vi "Water tank Sequence (1).vi"() -> ()   [LabVIEW 2023]
panel:
  out "Overhead Tank Chart":dbl(graph)
  out "Domestic Supply Chart":dbl(graph)
  out "Underground Tank Chart":dbl(graph)
  in  "Domestic Supply":bool
  in  "Overhead Tank":bool
  out "Domestic Supply":dbl(slide) scale=0.0..1000.0
  in  "Underground Tank":bool
  out "Overhead Tank":dbl(slide) scale=0.0..1000.0
  out "Underground Tank":dbl(slide) scale=0.0..5000.0
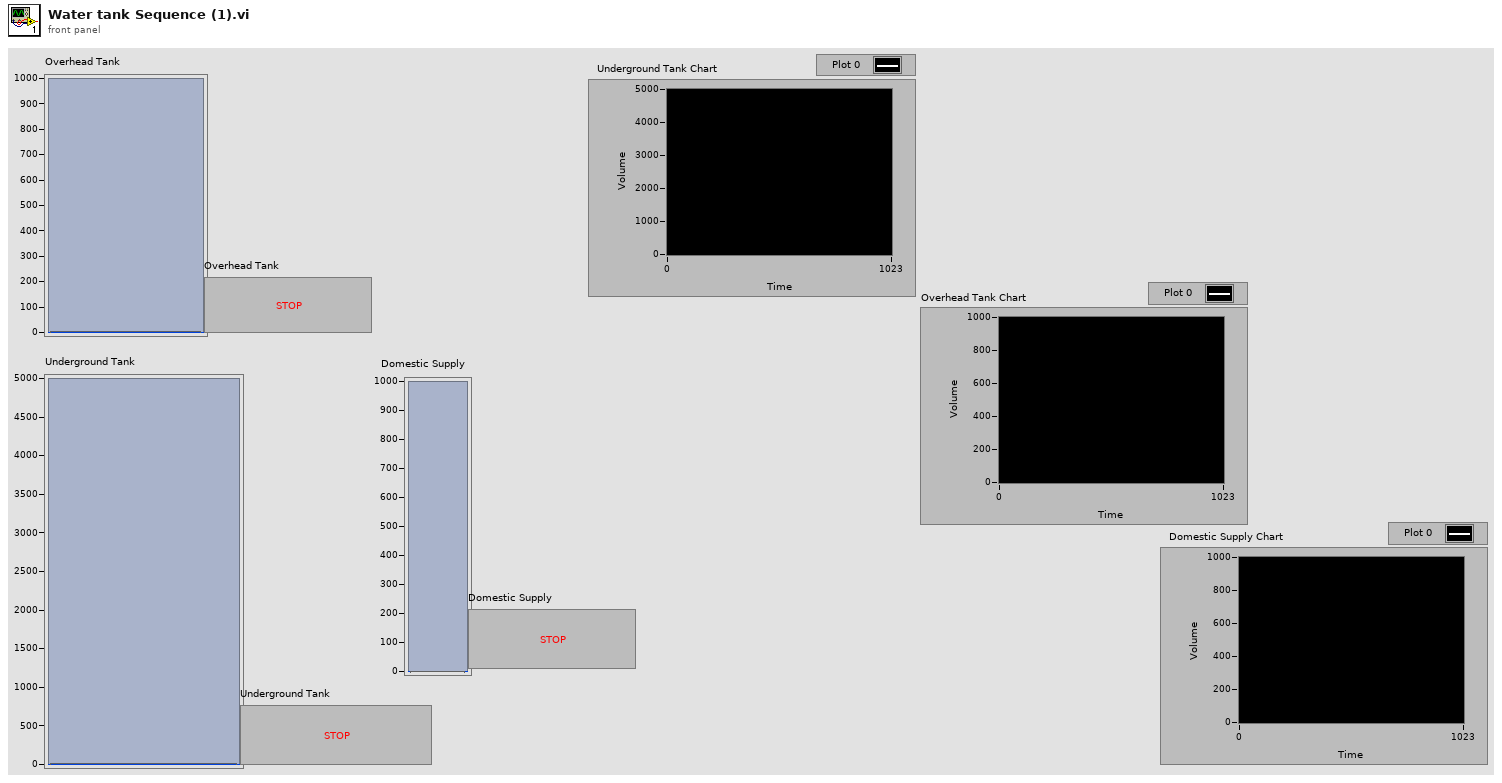
[diagram p1: front panel]
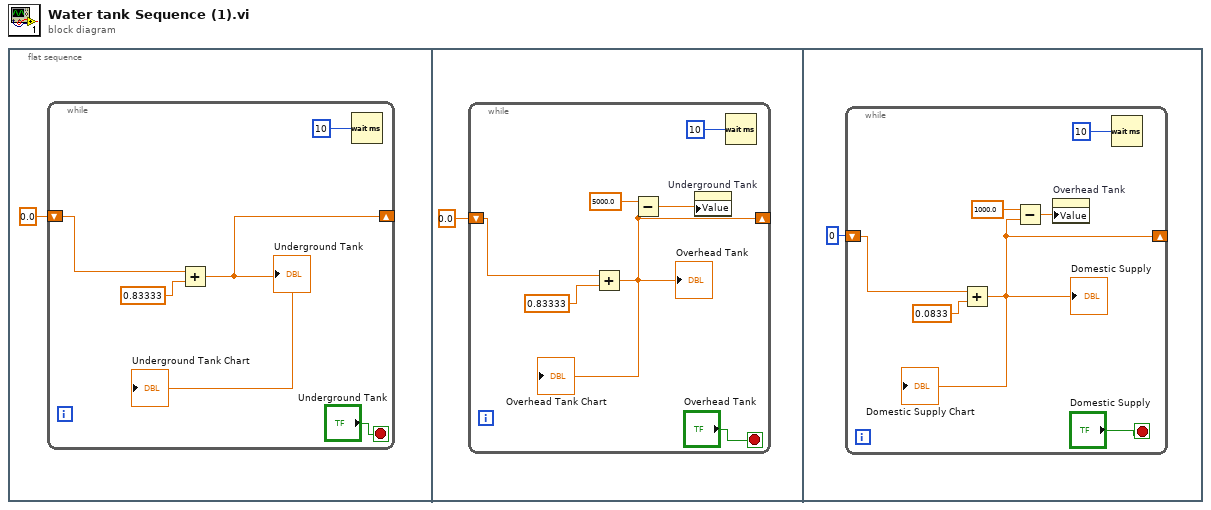
[diagram p0: block diagram]
diagram:
  n1 = flat-sequence {
    frame #0 {
      n2 = while {
        shift-right: [w2] -> _
        shift-left: 0.0 -> [w4]
        stop <- "Underground Tank" stop-if-true
        n3 = Add(x=w4, y=0.83333) -> (x+y=w2:dbl)
        "Underground Tank" <- w2
        "Underground Tank Chart" <- w2
        n4 = Wait (ms)(milliseconds to wait=u32 10) -> ()  [unwired: 1 out]
      }
    }
    frame #1 {
      n5 = while {
        shift-right: [w8] -> _
        shift-left: 0.0 -> [w12]
        stop <- "Overhead Tank" stop-if-true
        n6 = Add(x=w12, y=0.83333) -> (x+y=w8:dbl)
        "Overhead Tank" <- w8
        "Overhead Tank Chart" <- w8
        n7 = Subtract(x=5000.0, y=w8) -> (x-y=w11:dbl)
        n8 = property on="Underground Tank" class="Slide (strict)"("Value"=w11) -> ()  [unwired: 2 in, 2 out]
        n9 = Wait (ms)(milliseconds to wait=u32 10) -> ()  [unwired: 1 out]
      }
    }
    frame #2 {
      n10 = while {
        shift-right: [w17] -> _
        shift-left: 0 -> [w18]
        stop <- "Domestic Supply" stop-if-true
        n11 = Add(x=w18, y=0.0833) -> (x+y=w17:dbl)
        "Domestic Supply" <- w17
        "Domestic Supply Chart" <- w17
        n12 = Subtract(x=1000.0, y=w17) -> (x-y=w21:dbl)
        n13 = property on="Overhead Tank" class="Slide (strict)"("Value"=w21) -> ()  [unwired: 2 in, 2 out]
        n14 = Wait (ms)(milliseconds to wait=u32 10) -> ()  [unwired: 1 out]
      }
    }
  }
